vi "E364XA Commands.vi"(0 "VISA session":refnum<visa-resource-name>="COM3", 7 "Command":u16(ring) items=["Output Off", "Output On", "Output?", "Voltage Range Low", "Voltage Range High", "Voltage Range?", "Apply 12V, 1.5A", "Apply?", "Voltage 12V", "Voltage?", "Current 1.5A", "Current?", "Measure Voltage", "Measure Current", "Set RS232", "Set Remote Mode", "Set Local Mode", "System Error?", "*IDN?", "*RST", "Instrument Sel?", "Instrument Sel Out 1", "Instrument Sel Out 2", "Display Mode VI", "Display Mode VV", "Display Mode II", "Apply 0V, 0A"], 11 "error in (no error)":errorcluster) -> (4 "VISA session out":refnum<visa-resource-name>, 6 "Response":string, 8 "Num Resp":dbl, 13 "Bytes at port":u8, 14 "Bytes Read":u8, 15 "error out":errorcluster)   [LabVIEW 2010]
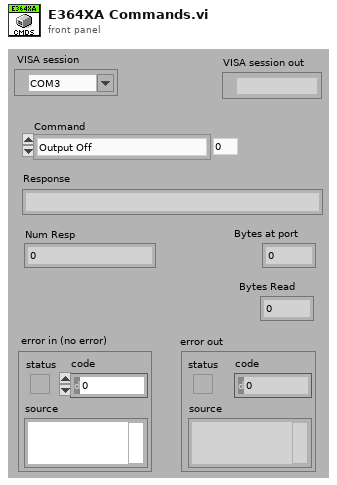
[diagram p1: front panel]
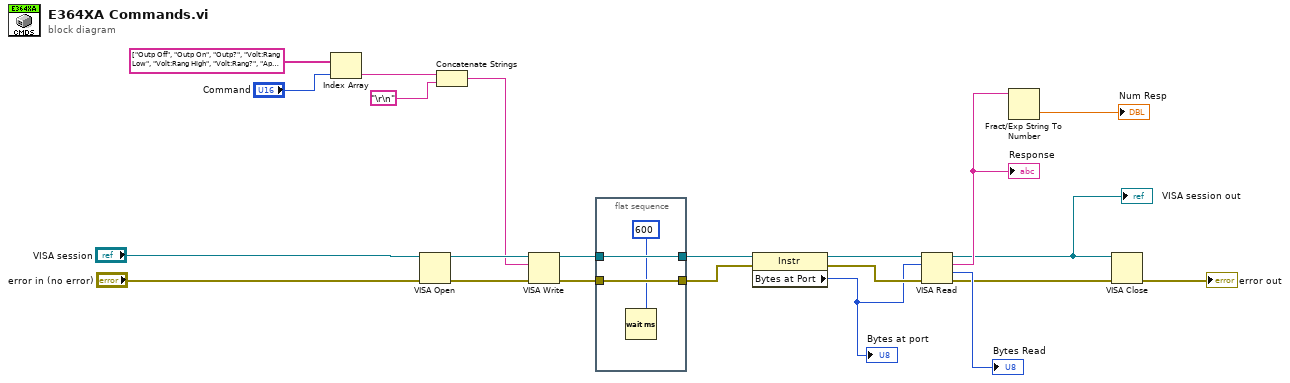
[diagram p0: block diagram]
diagram:
  n1 = Index Array(array=string[] ["Outp Off", "Outp On", "Outp?", "Volt:Rang Low", "Volt:Rang High", "Volt:Rang?", "Apply 12,1.5", "Apply?", "Volt 12", "Volt?", "Curr 1.5", "Curr?", "Meas:Volt?", "Meas:curr?", "Syst:Int RS232", "Syst:Rem", "Syst:Loc", "Syst:Err?", "*IDN?", "*RST", "INST:SEL?", "INST:SEL OUT1", "INST:SEL OUT2", "DISP:MODE VI", "DISP:MODE VV", "DISP:MODE II", "Apply 0,0"], index="Command") -> (element=w5:string)
  n2 = VISA Open(error in (no error)="error in (no error)", VISA resource name="VISA session") -> (VISA resource name=w21:refnum<visa-resource-name>, error out=w22:errorcluster)  [unwired: 3 in]
  n3 = Concatenate Strings(w5, "\r\n") -> (w19:string)
  n4 = VISA Write(VISA resource name=w21, write buffer=w19, error in (no error)=w22) -> (VISA resource name out=w13:refnum<visa-resource-name>, error out=w12:errorcluster)  [unwired: 1 out]
  n5 = flat-sequence {
    tunnel: [w25] -> w10
    tunnel: w13 -> [w25]
    tunnel: [w24] -> w11
    tunnel: w12 -> [w24]
    frame #0 {
      n6 = Wait (ms)(milliseconds to wait=600) -> ()  [unwired: 1 out]
    }
  }
  n7 = property class="Instr"(reference=w10, error in=w11) -> (reference out=w16:refnum<visa-resource-name>, error out=w15:errorcluster, "Bytes at Port"=w14:u32)
  "Bytes at port" <- w14
  n8 = VISA Read(VISA resource name=w16, byte count=w14, error in (no error)=w15) -> (VISA resource name out=w1:refnum<visa-resource-name>, read buffer=w9:string, return count=→"Bytes Read":u32, error out=w2:errorcluster)
  "Response" <- w9
  "VISA session out" <- w1
  n9 = Fract/Exp String To Number(string=w9) -> (number=→"Num Resp":dbl)  [unwired: 3 in, 1 out]
  n10 = VISA Close(VISA resource name=w1, error in (no error)=w2) -> (error out=→"error out":errorcluster)
